vi "PC_Lens_Calibration.vi"() -> ()   [LabVIEW 2017]
uses:
  <vilib>/vision/Calibration.llb/Distortion Model.ctl
  <vilib>/vision/Calibration.llb/Distortion Model Types.ctl
  <vilib>/vision/NI_Vision_Development_Module.lvlib
panel:
  in  "Grid Descriptor":cluster{"X Step":sgl, "Y Step":sgl, "Unit":T1}={"X Step"=10.0, "Y Step"=10.0, "Unit"=enum."Millimeter"}
  in  "Window Size (32x32)":cluster{"SizeX":i32, "SizeY":i32}={"SizeX"=32, "SizeY"=32}
  out "Image 2":T2(plugin-control)
  out "Image":T2(plugin-control)
  in  "File Path":path
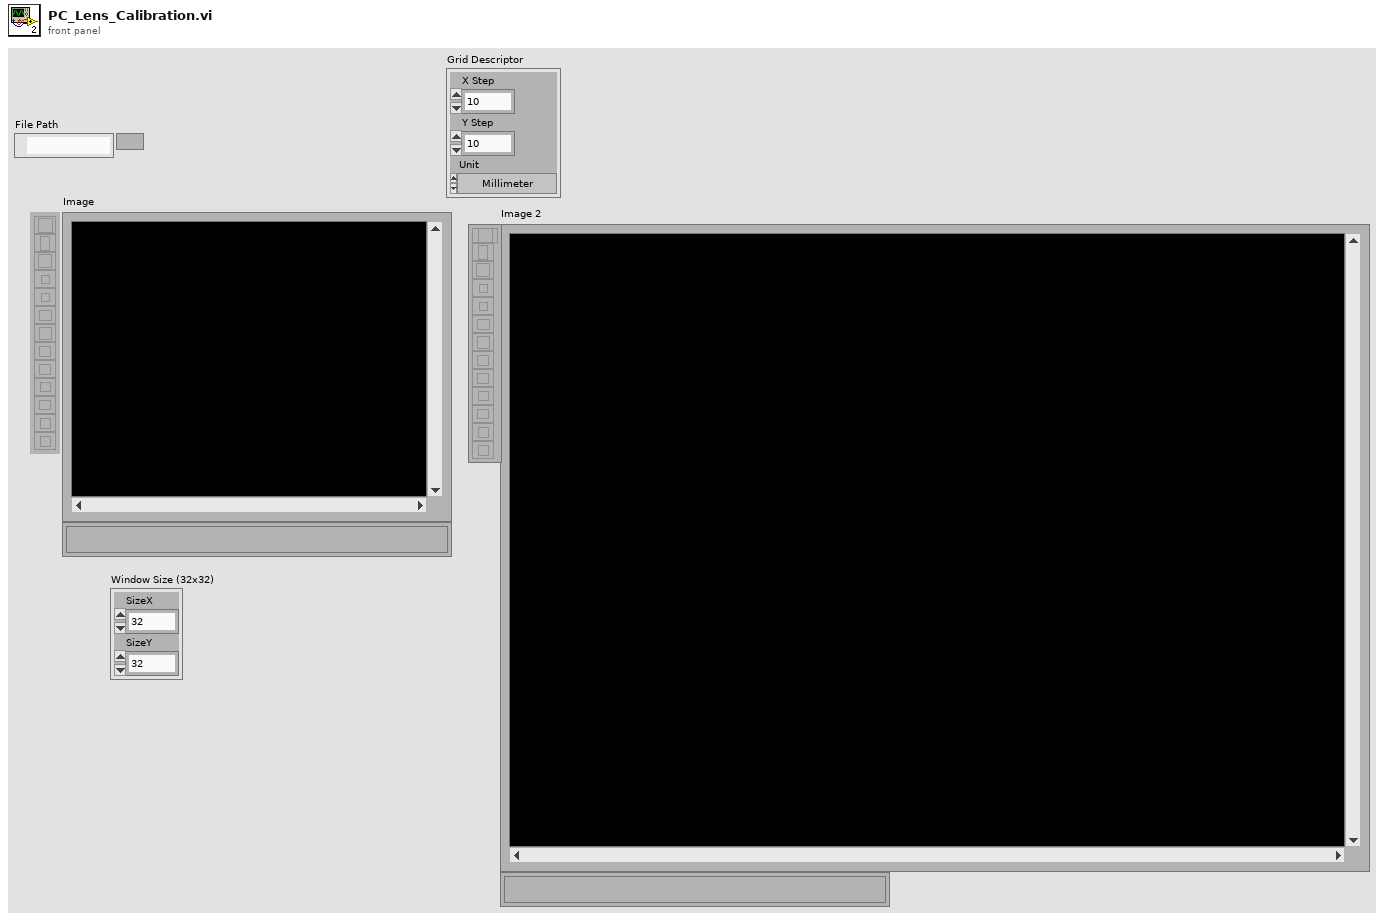
[diagram p1: front panel]
types:
  T1 = typedef "Image Unit" = enum32{"Undefined", "Angström", "Micrometer", "Millimeter", "Centimeter", "Meter", "Kilometer", "Microinch", "Inch", "Feet", "Nautical miles", "Standard miles", "Steps"}
  T2 = typedef "IMAQ Image.ctl" = refnum<image>
  T3 = typedef "Distortion Model.ctl" = cluster{"Distortion Model":T4, "Polynomial Model Setup":cluster{"Radial Coefficient":u32, "Tangential Coefficients ":bool}}
  T4 = typedef "Distortion Model Types.ctl" = i32
  T5 = typedef "Particle Parameters" = i32
  T6 = cluster{"Measurement Parameter":T5, "Range Lower Value":dbl, "Range Upper Value":dbl, "Range":bool, "Particle Parameters":bool}[]
  T7 = typedef "Calibration Reference Points.ctl" = cluster{"Pixel Coordinates":cluster{"X":dbl, "Y":dbl}[], "Real World Coordinates":cluster{"X":dbl, "Y":dbl}[], "Unit":T1, "Image Size":cluster{"X":u32, "Y":u32}}
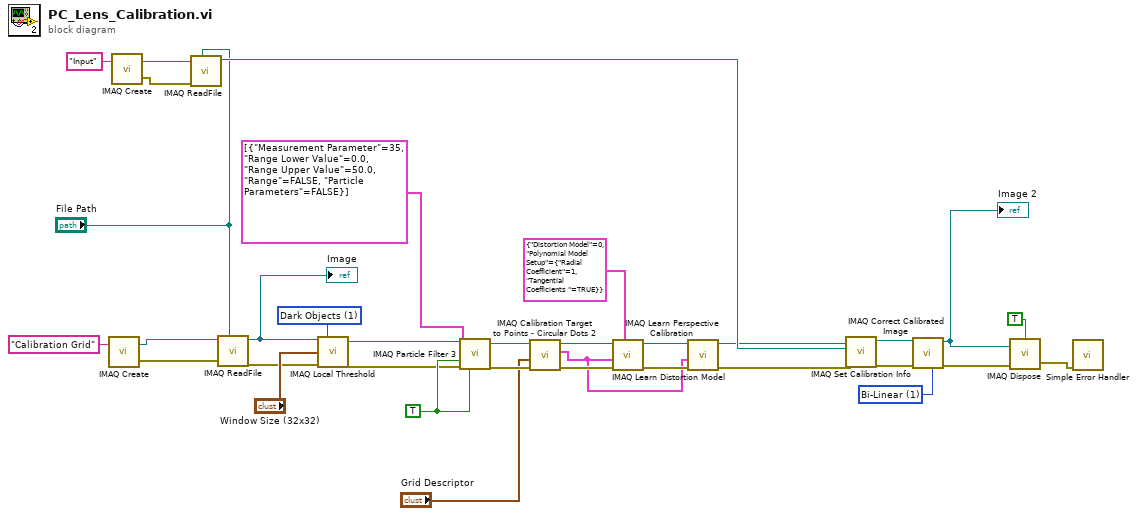
[diagram p0: block diagram]
diagram:
  w7 = u32 1 items=["Zero Order", "Bi-Linear", "Quadratic", "Cubic Spline"] ("Interpolation Type")
  w26 = TRUE ("Keep/Remove Particles (F)")
  w27 = u32 1 items=["Bright Objects", "Dark Objects"] ("Look For (Bright Objects)")
  n1 = call "IMAQ Create"("Image Name"="Calibration Grid") -> ("New Image"=w32:T2, "error out"=w33:errorcluster)  [unwired: 4 in]
  n2 = call "IMAQ Create"("Image Name"="Input") -> ("New Image"=w31:T2, "error out"=w34:errorcluster)  [unwired: 4 in]
  n3 = call "IMAQ ReadFile"("File Path"="File Path", "error in (no error)"=w34, "Image"=w31) -> ("Image Out"=w9:T2)  [unwired: 4 in, 4 out]
  n4 = call "IMAQ ReadFile"("File Path"="File Path", "error in (no error)"=w33, "Image"=w32) -> ("error out"=w24:errorcluster, "Image Out"=w5:T2)  [unwired: 4 in, 3 out]
  "Image" <- w5
  n5 = call "IMAQ Local Threshold"("Image Src"=w5, "Look For (Bright Objects)"=w27, "Window Size (32x32)"="Window Size (32x32)", "error in (no error)"=w24) -> ("Image Dst Out"=w23:T2, "error out"=w25:errorcluster)  [unwired: 10 in]
  n6 = call "IMAQ Particle Filter 3"("Image Src"=w23, "Selection Values"=T6 [{"Measurement Parameter"=35, "Range Lower Value"=0.0, "Range Upper Value"=50.0, "Range"=FALSE, "Particle Parameters"=FALSE}], "Keep/Remove Particles (F)"=w26, "error in (no error)"=w25, "Reject Border? (F)"=w26) -> ("Image Dst Out"=w15:T2, "error out"=w17:errorcluster)  [unwired: 8 in, 1 out]
  n7 = call "IMAQ Calibration Target to Points - Circular Dots 2"("error in (no error)"=w17, "Grid Descriptor"="Grid Descriptor", "Target Image"=w15) -> ("error out"=w18:errorcluster, "Reference Points"=w11:T7, "Target Image (dup)"=w14:T2)  [unwired: 6 in]
  n8 = call "IMAQ Learn Distortion Model"("Distortion Model Setup"=T3 {"Distortion Model"=0, "Polynomial Model Setup"={"Radial Coefficient"=1, "Tangential Coefficients "=TRUE}}, "error in (no error)"=w18, "Reference Points"=w11, "Calibration Template Image"=w14) -> ("error out"=w19:errorcluster, "Calibration Template Image Out"=w13:T2)  [unwired: 6 in]
  n9 = call "IMAQ Learn Perspective Calibration"("error in (no error)"=w19, "Reference Points"=w11, "Calibration Template Image"=w13) -> ("error out"=w2:errorcluster, "Calibration Template Image Out"=w1:T2)  [unwired: 7 in]
  n10 = call "IMAQ Set Calibration Info"("error in (no error)"=w2, "Image Dst"=w9, "Image Src"=w1) -> ("error out"=w20:errorcluster, "Calibrated Image"=w12:T2)  [unwired: 7 in]
  n11 = call "IMAQ Correct Calibrated Image"("Interpolation Type"=w7, "error in (no error)"=w20, "Image Src"=w12) -> ("error out"=w4:errorcluster, "Corrected Image"=w3:T2)  [unwired: 7 in]
  "Image 2" <- w3
  n12 = call "IMAQ Dispose"("All Images? (No)"=TRUE, "Image"=w3, "error in (no error)"=w4) -> ("error out"=w21:errorcluster)  [unwired: 3 in]
  n13 = call <vilib>:"Simple Error Handler.vi"("error in (no error)"=w21) -> ()  [unwired: 4 in, 5 out]
